vi "Example Arduino Blink LED.vi"(8 "Error In":errorcluster) -> (0 "Error Out":errorcluster)   [LabVIEW 2014]
panel:
  # "Output of generated code from this VI should be like:\n\n#include <ArduinoSTL.h>\n#include <vector>\n#include <ArduinoBasicFunctions.h>\nusing namespace std;\n\nvoid Blink_LED(){\n    bool wireUID_424_ = true;\n    bool wireUID_740_ = true;\n    long wireUID_705_ = 3;\n    long wireUID_652_ = 2;\n    pinMode(wireUID_652_,wireUID_740_?OUTPUT:INPUT);\n    pinMode(wireUID_705_,wireUID_740_?OUTPUT:INPUT);\n    /***** BEGIN WhileLoop ********/\n    vector<bool> feedbackNode_615;\n    bool feedbackNodeInitBool_615 = true;\n    \n    bool wireUID_430_ = false; //LoopEndRef.\n    int iteratorUID_289 = 0; //loop iterator\n    do{\n     //shift register init and get front value\n        bool wireUID_317_;\n        bool wireUID_642_;\n        long wireUID_1157_ = 2;\n        long wireUID_921_ = 3;\n        long wireUID_426_ = 220;\n        if (feedbackNodeInitBool_615){\n            feedbackNode_615.push_back(wireUID_424_);\n            feedbackNodeInitBool_615 = false;\n        }\n        wireUID_642_ = feedbackNode_615.front(); feedbackNode_615.erase(feedbackNode_615.begin());\n        delay(wireUID_426_);\n        wireUID_317_ = !wireUID_642_;\n        digitalWrite(wireUID_921_,wireUID_642_?HIGH:LOW);\n        /* Don't know how to translate class \"Generic ->GObject ->Node\": \"\" */\n        digitalWrite(wireUID_1157_,wireUID_317_?HIGH:LOW);\n        feedbackNode_615.push_back(wireUID_317_);\n         //C code\n        \n         //output assgn.\n        iteratorUID_289++; //iterator increment\n    }while(!wireUID_430_); //negation because in LabVIEW it is when stop (oposite)\n    /****** END WhileLoop */\n    \n}\n\nvoid setup(){}\nvoid loop(){\n    Blink_LED();\n}"
  # "Good result, LED on pin 3 ON:"
  # "after few hundred ms switch to pin 2 LED ON"
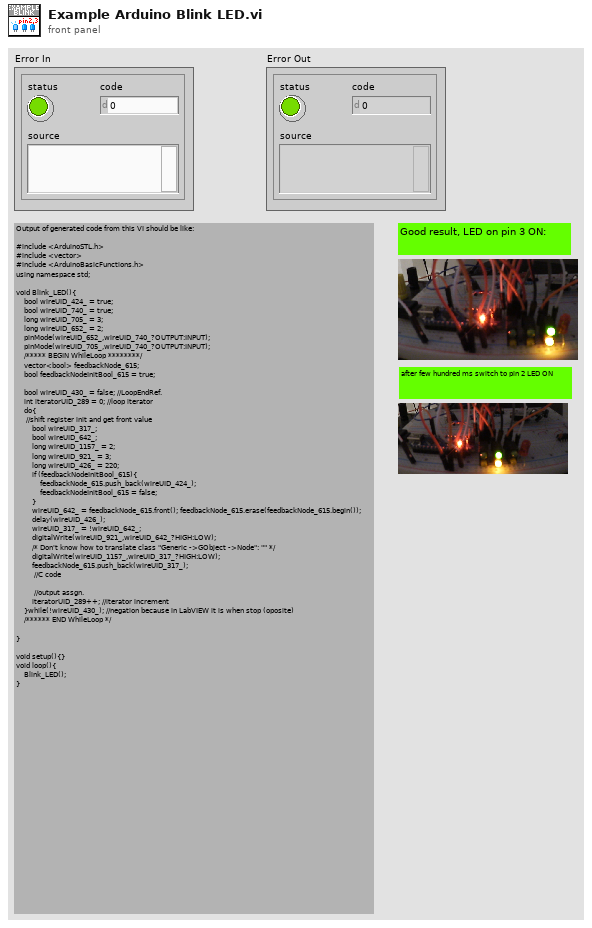
[diagram p1: front panel]
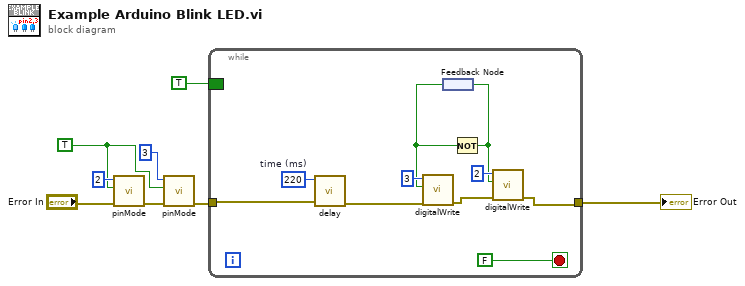
[diagram p0: block diagram]
diagram:
  w2 = TRUE
  n1 = call "pinMode.vi"("Error In"="Error In", "output?"=w2, "pin number"=2) -> ("Error Out"=w6:errorcluster)  [unwired: 8 in]
  n2 = call "pinMode.vi"("Error In"=w6, "output?"=w2, "pin number"=3) -> ("Error Out"=w7:errorcluster)  [unwired: 8 in]
  n3 = while {
    tunnel: w7 -> [w18]
    tunnel: [w15] -> w8
    border: TRUE -> [_]
    stop <- FALSE stop-if-true
    w16 = 220  # time (ms)
    n4 = call "delay.vi"("Error In"=w18, "time (ms)"=w16) -> ("Error Out"=w17:errorcluster)  [unwired: 9 in]
    n5 = feedback #1() -> (w10:bool)
    n6 = call "digitalWrite.vi"("Error In"=w17, "value"=w10, "pin number"=3) -> ("Error Out"=w11:errorcluster)  [unwired: 8 in]
    n7 = Not(x=w10) -> (.not. x?=w9:bool)
    n8 = feedback-in #1(w9) -> ()
    n9 = call "digitalWrite.vi"("Error In"=w11, "value"=w9, "pin number"=2) -> ("Error Out"=w15:errorcluster)  [unwired: 8 in]
  }
  "Error Out" <- w8
